vi "WriteStringUART.vi"(8 "error in":errorcluster, 10 "String":string, 11 "FPGA VI Reference In":refnum<k20>) -> (0 "error out":errorcluster, 3 "FPGA VI ReferenceOut":refnum<k20>)   [LabVIEW 2012]
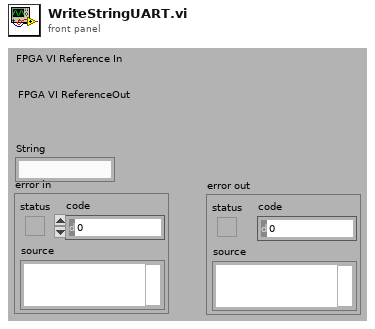
[diagram p1: front panel]
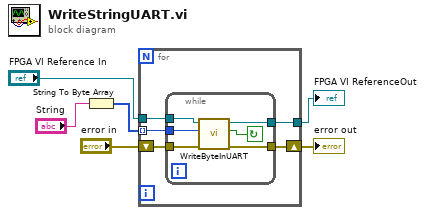
[diagram p0: block diagram]
diagram:
  n1 = String To Byte Array(string="String") -> (unsigned byte array=w5:u8[])
  n2 = for {
    tunnel: "FPGA VI Reference In" -> [w11]
    tunnel: [w10] -> w1
    tunnel: w5 -> [w9] mode=indexing
    shift-right: [w7] -> w3
    shift-left: "error in" -> [w8]
    n3 = while {
      tunnel: w11 -> [w17]
      tunnel: [w16] -> w10
      tunnel: w9 -> [w15]
      tunnel: w8 -> [w14]
      tunnel: [w13] -> w7
      stop <- w12 continue-if-true
      n4 = call "WriteByteInUART.vi"("error  in"=w14, "Byte Value"=w15, "FPGA VI Reference In"=w17) -> ("error out"=w13:errorcluster, "Overflow?"=w12:bool, "FPGA VI Reference Out"=w16:refnum<k20>)  [unwired: 5 in]
    }
  }
  "error out" <- w3
  "FPGA VI ReferenceOut" <- w1
